vi "Post Install Script.vi"() -> ()   [LabVIEW 2013]
uses:
  <vilib>/Utility/sysdir.llb/System Directory Type.ctl
panel:
  out "error out":errorcluster
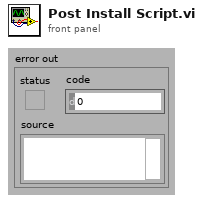
[diagram p1: front panel]
types:
  T1 = typedef "System Directory Type.ctl" = i32
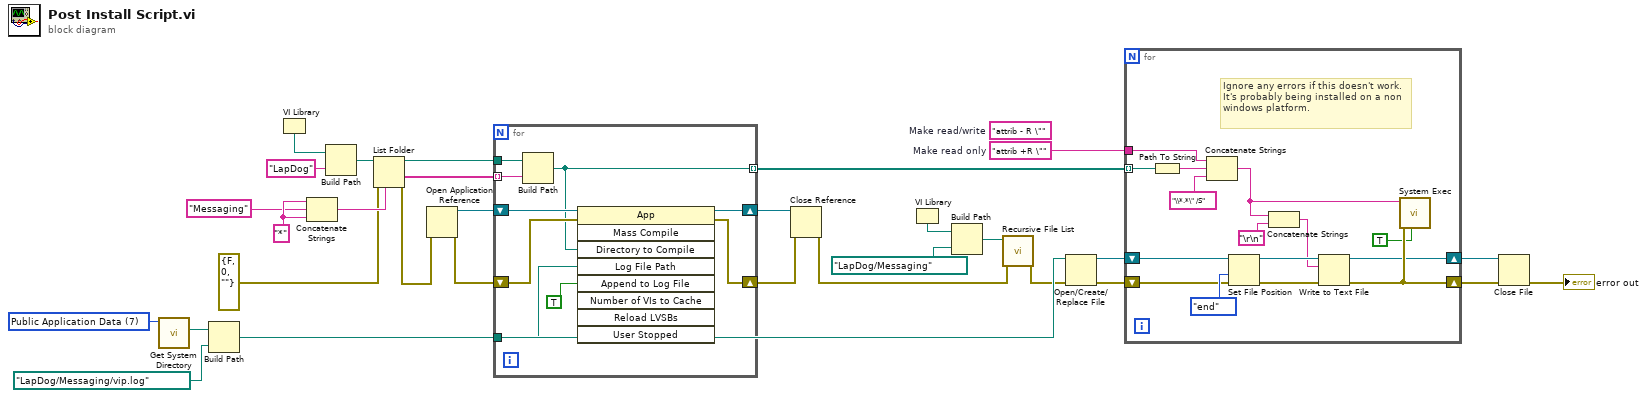
[diagram p0: block diagram]
diagram:
  (unwired) "attrib - R \""  # Make read/write
  w15 = "attrib +R \""  # Make read only
  w29 = T1 7 items=["User Home", "User Desktop", "User Documents", "User Application Data", "User Preferences", "User Temporary", "Public Documents", "Public Application Data", "Public Preferences", "System Core Libraries", "System Installed Libraries", "Application Files", "Boot Volume Root"] ("system directory type")
  w22 = "*"
  n1 = call <vilib>:"Get System Directory.vi"("system directory type"=w29) -> ("system directory"=w30:path)  [unwired: 10 in]
  n2 = Build Path(base path=w30, name or relative path=path "LapDog/Messaging/vip.log" ("Log File Path")) -> (appended path=w12:path)
  n3 = VI Library() -> (path=w20:path)
  n4 = Concatenate Strings(w22, "Messaging" ("Path Filter"), w22) -> (w21:string)
  n5 = Build Path(base path=w20, name or relative path="LapDog") -> (appended path=w27:path)
  n6 = List Folder(path=w27, pattern=w21, error in=errorcluster {"status"=FALSE, "code"=0, "source"=""}) -> (path out=w28:path, folder names=w5:string[], error out=w13:errorcluster)  [unwired: 1 in, 1 out]
  n7 = Open Application Reference(8:w13) -> (0:w24:errorcluster, 3:w23:refnum<vi>)  [unwired: 3 in]
  n8 = for {
    tunnel: w5 -> [w35] mode=indexing
    shift-right: [w38] -> w26
    shift-left: w24 -> [w39]
    shift-right: [w36] -> w25
    shift-left: w23 -> [w37]
    tunnel: w28 -> [w34]
    tunnel: w12 -> [w33]
    tunnel: [w31] -> w4 mode=indexing
    n9 = Build Path(base path=w34, name or relative path=w35) -> (appended path=w31:path)
    n10 = invoke class="App" method="Mass Compile"(reference=w37, error in=w39, "Directory to Compile"=w31, "Log File Path"=w33, "Append to Log File"=TRUE) -> (reference out=w36:refnum<vi>, error out=w38:errorcluster)  [unwired: 4 in, 7 out]
  }
  n11 = Close Reference(reference=w25, error in (no error)=w26) -> (error out=w17:errorcluster)
  n12 = VI Library() -> (path=w3:path)
  n13 = Build Path(base path=w3, name or relative path=path "LapDog/Messaging") -> (appended path=w1:path)
  n14 = call <vilib>:"Recursive File List.vi"("error in (no error)"=w17, "Folder Path"=w1) -> ("error out"=w10:errorcluster)  [unwired: 5 in, 4 out]
  n15 = Open/Create/Replace File(file path (use dialog)=w12, error in=w10) -> (refnum out=w11:refnum<file>, error out=w9:errorcluster)  [unwired: 4 in, 1 out]
  n16 = for {
    tunnel: w4 -> [w54] mode=indexing
    shift-right: [w53] -> w8
    shift-left: w9 -> [w40]
    tunnel: w15 -> [w49]
    shift-right: [w47] -> w6
    shift-left: w11 -> [w52]
    # "Ignore any errors if this doesn't work.  It's probably being installed on a non windows platform."
    n17 = Path To String(path=w54) -> (string=w51:string)
    n18 = Concatenate Strings(w49, w51, "\\*.*\" /S" ("string")) -> (w48:string)
    n19 = Set File Position(refnum=w52, from (0:start)=enum16{"start", "end", "current"}."end", error in=w40) -> (refnum out=w44:refnum<file>, error out=w45:errorcluster)  [unwired: 1 in]
    n20 = Concatenate Strings(w48, "\r\n") -> (w42:string)
    n21 = Write to Text File(file (use dialog)=w44, text=w42, error in=w45) -> (refnum out=w47:refnum<file>, error out=w53:errorcluster)  [unwired: 1 in, 1 out]
    n22 = call <vilib>:"System Exec.vi"("run minimized? (F)"=TRUE, "error in (no error)"=w53, "command line"=w48) -> ()  [unwired: 5 in, 4 out]
  }
  n23 = Close File(refnum=w6, error in=w8) -> (error out=→"error out":errorcluster)  [unwired: 1 out]
